vi "CE Measure.vi"(5 "PJVS setup":T1={"PJVS type"=enum."AC-supraVOLTcontrol", "Status Refnum"=refnum, "AC-supraVOLTcontrol"={"IP address:port (0.0.0.0:0000)"="0.0.0.0:0000", "Timeouts"={"TCP Read & Write (ms)"=7000, "Sensors readout"=5000, "PJVS setup"=10000, "Nullmeter readout"=5000, "Multiplexer setup"=3000, "57XX setup"=15000, "Generator setup"=5000, "Synthesizer setup"=3000, "Sampler readout"=10000}, "Simulation mode"=FALSE, "Debug mode"=FALSE}, "NPL bias source"={"DataSocketCluster"={"Server Machine"="CZC", "Client Machine"="localhost", "Data"="P2", "TimeStamp"=0.0, "Count"=1, "Target Process"="General Server"}}, "Manual PJVS"={"PJVS frequency (Hz)"=0.0, "Reference voltages (V)"=[], "File with PJVS voltages"=path ""}, "VTT PJVS"={"some VTT only property"=""}} {"NPL bias source"."DataSocketCluster"."TimeStamp" format="%.2f"}, 6 "AC sync source":T5, 7 "figure prefix ()":string, 8 "error in":errorcluster, 9 "CE measurement":T7={"Signal frequencies (Hz) T"=[1000.0], "Signal amplitudes (V) T"=[0.707], "Sampling frequencies (Hz) T"=[10000000.0], "Record lengths (multiples of periods) T"=[10000.0], "TWM data root directory"=path "", "TWM mreasurements directories"=[], "Calculate RMS from samples"=FALSE, "Algorithm to use"="TWM-WFFT", "Quantity to read"="TWM-WFFT", "Settle down after AC source change (s) T"=1.0, "Skip PJVS setup"=FALSE, "Measurement template file"=path "", "Row of START keyword T"=0, "Row of STOP keyword T"=0, "Measurement template line T"=[], "Switch position T"=[10000.0], "FR fit mat file T"=path "", "Recalculate-skip already calculated"=FALSE} {"Switch position T" format="%#_3p"; "Record lengths (multiples of periods) T" format="%#_3p"; "Sampling frequencies (Hz) T" format="%#_3p"; "Signal amplitudes (V) T" format="%#_3p"; "Signal frequencies (Hz) T" format="%#_3p"}, 10 "AC Source":T5, 11 "Common properties":T8={"Measurement status ref"=refnum, "TWM Status ref"=refnum, "Abort ref"=refnum, "Skip waiting ref"=refnum, "GNU Octave path"=path "C:/Program Files/GNU Octave/Octave-6.2.0/mingw64/bin", "TWM+QWTB path"=path "C:/Users/labina/Desktop/TWM-1.8.7.0-full/octprog", "lvlib path"=path "D:/martin/WAC/WACsw - github/control_software/Filter function meter/external libraries/GOLPI 0.7.3.1 source distribution LV 20.0 32 bit/lv_proc.dll", "TWM pipe"="\\\\.\\pipe\\TWM:server", "PJVS status ref"=refnum, "WAC path"=path ""}) -> (0 "error out":errorcluster)   [LabVIEW 2020]
doc: "Main VI to run cable error measurement. Setup devices, run loop for all freuencies, stop devices."
uses:
  General AC source/Type definitions/AC Source.ctl
  General AC source/Type definitions/AC Source type.ctl
  Utilities/Type definitions/Common properties.ctl
  Type definitions/CE measurement.ctl
  <vilib>/Utility/NIReport.llb/NI_report.lvclass
  General PJVS driver/Type definitions/PJVS.ctl
  General PJVS driver/Type definitions/PJVS Type.ctl
  external libraries/acsvcontrol-driver/Public/Type Definitions/Timeouts.ctl
  external libraries/JV modified NPL Bias source/DataSocketCluster external.ctl
  <vilib>/Utility/error.llb/DialogType.ctl
  external libraries/TWM-1.8.7.0-client/TWM Client.lvlib
  external libraries/acsvcontrol-driver/ACSVcontrol-driver.lvlib
panel:
  out "NI_report":refnum<class "NI_report.lvclass">
  out "previous TWM result value":dbl
  out "previous AC source amplitude":dbl=nan format="%#_13g"
  out "previous AC source frequency":dbl=nan format="%#_13g"
  out "figure reference out":refnum<vi>
  out "TWM handle":i32
  out "figure queue":refnum<queue>
  out "graph x axis":dbl[](array[numeric])
  out "graph y axis":dbl[](array[numeric])
  out "ratio chart":cluster{dbl[], dbl[]}(graph)
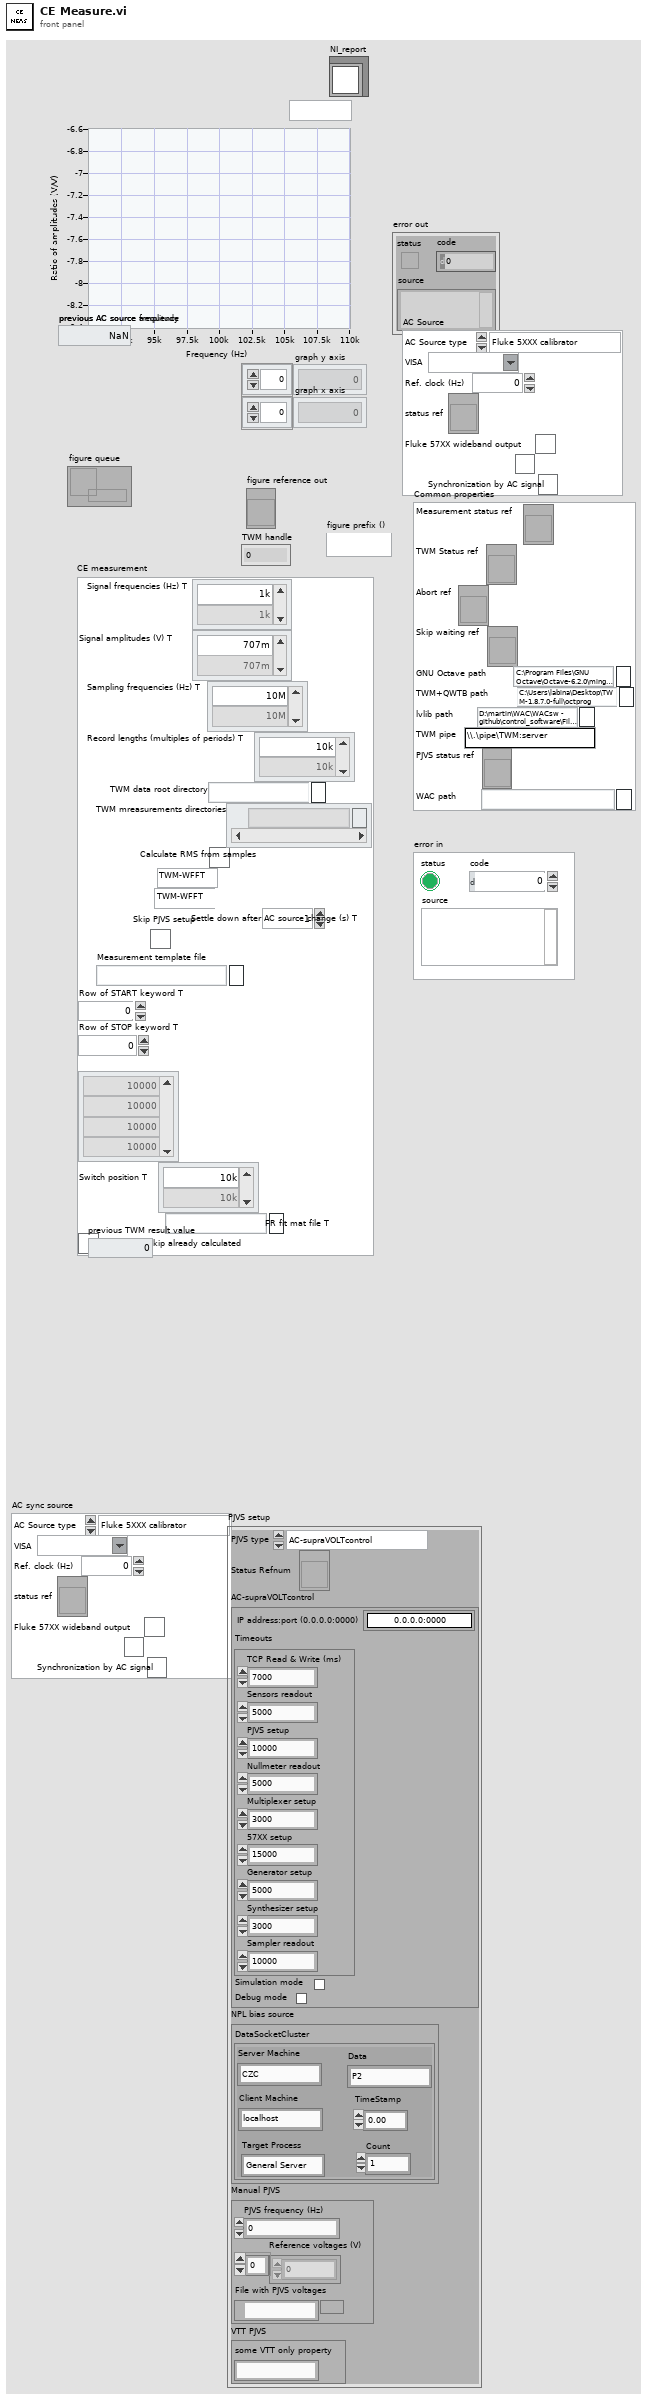
[diagram p1: front panel]
types:
  T1 = typedef "PJVS.ctl" = cluster{"PJVS type":T2, "Status Refnum":refnum<vi>, "AC-supraVOLTcontrol":cluster{"IP address:port (0.0.0.0:0000)":string, "Timeouts":T3, "Simulation mode":bool, "Debug mode":bool}, "NPL bias source":cluster{"DataSocketCluster":T4}, "Manual PJVS":cluster{"PJVS frequency (Hz)":dbl, "Reference voltages (V)":dbl[], "File with PJVS voltages":path}, "VTT PJVS":cluster{"some VTT only property":string}}
  T2 = typedef "PJVS Type.ctl" = enum16{"AC-supraVOLTcontrol", "JV modified NPL bias control", "Manual PJVS", "VTT PJVS"}
  T3 = typedef "ACSVcontrol-driver.lvlib/Timeouts.ctl" = cluster{"TCP Read & Write (ms)":i32, "Sensors readout":i32, "PJVS setup":i32, "Nullmeter readout":i32, "Multiplexer setup":i32, "57XX setup":i32, "Generator setup":i32, "Synthesizer setup":i32, "Sampler readout":i32}
  T4 = typedef "DataSocketCluster external.ctl" = cluster{"Server Machine":string, "Client Machine":string, "Data":string, "TimeStamp":dbl, "Count":i32, "Target Process":string}
  T5 = typedef "AC Source.ctl" = cluster{"AC Source type":T6, "VISA":refnum<visa-resource-name>, "Ref. clock (Hz)":dbl, "status ref":refnum<vi>, "Fluke 57XX wideband output":bool, "Fluke 57XX ignore errors":bool, "Synchronization by AC signal":bool}
  T6 = typedef "AC Source type.ctl" = enum16{"Fluke 5XXX calibrator", "Tektronix AFG3000 series", "dummy", "Agilent 331xxA to 332xxA", "Agilent 335xxA to 336xxA"}
  T7 = typedef "CE measurement.ctl" = cluster{"Signal frequencies (Hz) T":dbl[], "Signal amplitudes (V) T":dbl[], "Sampling frequencies (Hz) T":dbl[], "Record lengths (multiples of periods) T":dbl[], "TWM data root directory":path, "TWM mreasurements directories":path[], "Calculate RMS from samples":bool, "Algorithm to use":string, "Quantity to read":string, "Settle down after AC source change (s) T":dbl, "Skip PJVS setup":bool, "Measurement template file":path, "Row of START keyword T":i32, "Row of STOP keyword T":i32, "Measurement template line T":i32[], "Switch position T":dbl[], "FR fit mat file T":path, "Recalculate-skip already calculated":bool}
  T8 = typedef "Common properties.ctl" = cluster{"Measurement status ref":refnum<vi>, "TWM Status ref":refnum<vi>, "Abort ref":refnum<vi>, "Skip waiting ref":refnum<vi>, "GNU Octave path":path, "TWM+QWTB path":path, "lvlib path":path, "TWM pipe":string, "PJVS status ref":refnum<vi>, "WAC path":path}
  T9 = typedef "DialogType.ctl" = u16
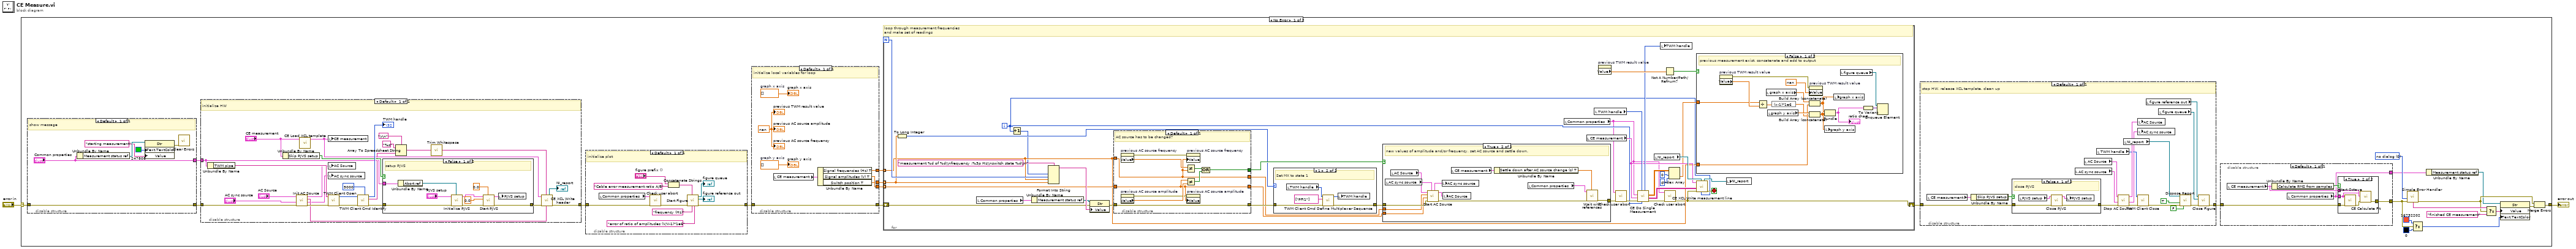
[diagram p0: block diagram]
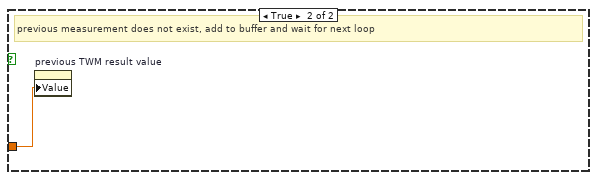
[diagram p3: hidden frame]
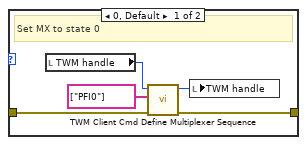
[diagram p5: hidden frame]
diagram:
  n1 = case shown="No Error" "error in" {
    selector: "error in" -> [w3 w206]
    tunnel: [w10 w206] -> w2
    frame No Error {
      w12 = T9 0 items=["no dialog", "OK message", "continue or stop message", "OK message + warnings", "continue/stop + warnings"] ("type of dialog (OK msg:1)")
      n2 = disable-structure shown="Default" {
        disable-tunnel: w3 -> [w58]
        disable-tunnel: [w58] -> w24
        disable-tunnel: ["Common properties"] -> w23
        frame Enabled {
          # "show message"
          n3 = Unbundle By Name("Common properties") -> ("Measurement status ref"=w61:refnum<vi>)
          n4 = property class="Str"(reference=w61, "Text.TextColor"=u32 247808 ("Text.Text Colors:Text Color"), "Value"="starting measurement") -> (error out=w62:errorcluster)  [unwired: 1 in, 1 out]
          n5 = call <vilib>:"Clear Errors.vi"("error in (no error)"=w62) -> ()  [unwired: 5 in, 2 out]
        }
      }
      n6 = disable-structure shown="Default" {
        disable-tunnel: [w180] -> w26
        disable-tunnel: w24 -> [w186]
        disable-tunnel: w23 -> [w170]
        frame Enabled {
          # "initialize HW"
          n7 = Unbundle By Name(w170) -> ("TWM pipe"=w189:string)
          n8 = Unbundle By Name("CE measurement") -> ("Skip PJVS setup"=w185:bool)
          n9 = call "Init AC Source.vi"("error in (no error)"=w186, "AC sync source"="AC sync source", "AC source"="AC Source") -> ("error out"=w190:errorcluster, "AC sync source out"=w171:T5, "Init status"=w179:string, "AC source out"=w187:T5)  [unwired: 5 in]
          n10 = call "CE Load XCL template.vi"("CE measurement"="CE measurement") -> ("CE measurement out"=w182:T7)  [unwired: 9 in, 1 out]
          n11 = local write "CE measurement"(w182) -> ()
          n12 = local write "AC Source"(w187) -> ()
          n13 = local write "AC sync source"(w171) -> ()
          n14 = call "TWM Client Open.vi"("error in"=w190, "pipe name"=w189) -> ("error out"=w193:errorcluster, "handle out"=w194:i32)  [unwired: 8 in]
          n15 = call "TWM Client Cmd Identify.vi"("timeout [ms]"=5000, "error in"=w193, "handle"=w194) -> ("error out"=w184:errorcluster, "channel idns"=w176:string[], "handle out"=→"TWM handle":i32)  [unwired: 5 in, 1 out]
          n16 = case shown="False" w185 {
            tunnel: [w200 w205] -> w181
            tunnel: w184 -> [w201 w205]
            tunnel: w170 -> [w197 _]
            frame False {
              # "setup PJVS"
              n17 = Unbundle By Name(w197) -> ("Abort ref"=w196:refnum<vi>)
              n18 = call "Initialize PJVS.vi"("Abort Refnum"=w196, "error in (no error)"=w201, "PJVS setup"="PJVS setup") -> ("error out"=w202:errorcluster, "PJVS setup out"=w198:T1)  [unwired: 7 in]
              n19 = call "Start PJVS.vi"("Requested PJVS frequency (Hz)"=0.0, "error in (pass through)"=w202, "Maximal signal amplitude (V)"=0.0, "PJVS setup"=w198) -> ("error out"=w200:errorcluster, "PJVS setup out"=w195:T1)  [unwired: 3 in, 3 out]
              n20 = local write "PJVS setup"(w195) -> ()
            }
            frame True {
            }
          }
          n21 = Array To Spreadsheet String(delimiter (Tab)="\r\n", array=w176, 3:"%s" ("format string")) -> (spreadsheet string=w178:string)
          n22 = call <vilib>:"Trim Whitespace.vi"("string"=w178) -> ("trimmed string"=w174:string)  [unwired: 1 in]
          n23 = call "CE XCL Write header.vi"("AC source idn"=w179, "Digitizer idn"=w174, "error in (no error)"=w181, "CE measurement"=w182) -> ("error out"=w180:errorcluster, "NI_report out"=→"NI_report":refnum<class "NI_report.lvclass">)  [unwired: 6 in]
        }
      }
      n24 = disable-structure shown="Default" {
        disable-tunnel: w26 -> [w56]
        disable-tunnel: [w46] -> w22
        frame Enabled {
          # "initialize plot"
          n25 = local read "Common properties"() -> (w51:T8)
          n26 = call "Check user abort.vi"("error in (no error)"=w56, "Common properties"=w51) -> ("error out"=w55:errorcluster)  [unwired: 9 in]
          n27 = Concatenate Strings("figure prefix ()", "Cable error measurement ratio A/B" ("Plot name (sampled signal)")) -> (w47:string)
          n28 = call "Start Figure.vi"("Y scale label (amplitude (V))"="error of ratio of amplitudes (V/V-1)*1e6", "X scale label (time(s))"="frequency (Hz)", "Plot name (sampled signal)"=w47, "error in (no error)"=w55) -> ("error out"=w46:errorcluster, "figure reference out"=→"figure reference out":refnum<vi>, "queue out"=→"figure queue":refnum<queue>)  [unwired: 5 in]
        }
      }
      n29 = disable-structure shown="Default" {
        disable-tunnel: [w45] -> w21
        disable-tunnel: w22 -> [w45]
        disable-tunnel: [w40] -> w6
        disable-tunnel: [w39] -> w5
        disable-tunnel: [w38] -> w4
        frame Enabled {
          w42 = dbl[] []  # graph y axis
          w43 = dbl[] []  # graph x axis
          w44 = nan ("previous TWM result value")
          # "initialize local variables for loop"
          n30 = local read "CE measurement"() -> (w41:T7)
          n31 = Unbundle By Name(w41) -> ("Signal frequencies (Hz) T"=w40:dbl[], "Signal amplitudes (V) T"=w39:dbl[], "Switch position T"=w38:dbl[])
          "previous AC source frequency" <- w44
          "previous AC source amplitude" <- w44
          "previous TWM result value" <- w44
          "graph y axis" <- w42
          "graph x axis" <- w43
        }
      }
      n32 = for {
        N -> [w96]
        shift-right: [w64] -> w25
        shift-left: w21 -> [w95]
        tunnel: w6 -> [w72] mode=indexing
        tunnel: w5 -> [w84] mode=indexing
        tunnel: w4 -> [w81] mode=indexing
        i -> [w67]
        stop <- w75 stop-if-true
        # "loop through measurement frequencies\nand make set of readings"
        n33 = To Long Integer(number=w81) -> (32bit integer=w80:i32)
        n34 = local read "Common properties"() -> (w93:T8)
        n35 = Increment(x=w67) -> (x+1=w66:i32)
        n36 = Unbundle By Name(w93) -> ("Measurement status ref"=w94:refnum<vi>)
        n37 = Format Into String(format string="measurement %d of %d\\nfrequency :%3p Hz\\nswitch state %d\\n", w66, w96, w72, w81) -> (resulting string=w97:string)  [unwired: 2 in, 1 out]
        n38 = property class="Str"(reference=w94, error in=w95, "Value"=w97) -> (error out=w87:errorcluster)  [unwired: 1 out]
        n39 = disable-structure shown="Default" {
          disable-tunnel: w84 -> [w100]
          disable-tunnel: w72 -> [w99]
          disable-tunnel: [w106] -> w85
          disable-tunnel: w87 -> [w106]
          disable-tunnel: [w103] -> w88
          disable-tunnel: [w100] -> w83
          disable-tunnel: [w99] -> w82
          frame Enabled {
            # "AC source has to be changed?"
            n40 = property on="previous AC source frequency" class="DigNum (strict)"() -> (error out=w101:errorcluster, "Value"=w108:dbl)  [unwired: 2 in, 1 out]
            n41 = property on="previous AC source amplitude" class="DigNum (strict)"() -> (error out=w102:errorcluster, "Value"=w107:dbl)  [unwired: 2 in, 1 out]
            n42 = Not Equal?(x=w108, y=w99) -> (x != y?=w104:bool)
            n43 = Not Equal?(x=w100, y=w107) -> (x != y?=w105:bool)
            n44 = property on="previous AC source frequency" class="DigNum (strict)"(error in=w101, "Value"=w99) -> ()  [unwired: 1 in, 2 out]
            n45 = property on="previous AC source amplitude" class="DigNum (strict)"(error in=w102, "Value"=w100) -> ()  [unwired: 1 in, 2 out]
            n46 = Compound Arithmetic op=OR(w104, w105) -> (w103:bool)
          }
        }
        n47 = case shown="1" w80 {
          tunnel: w85 -> [w138 w143]
          tunnel: [w137 w142] -> w86
          frame 0, Default {
            # "Set MX to state 0"
            n48 = local read "TWM handle"() -> (w140:i32)
            n49 = call "TWM Client Cmd Define Multiplexer Sequence.vi"("error in"=w138, "sequence item strings"=string[] ["PFI0"], "handle"=w140) -> ("error out"=w137:errorcluster, "handle out"=w141:i32)  [unwired: 7 in]
            n50 = local write "TWM handle"(w141) -> ()
          }
          frame 1 {
            # "Set MX to state 1"
            n51 = local read "TWM handle"() -> (w145:i32)
            n52 = call "TWM Client Cmd Define Multiplexer Sequence.vi"("error in"=w143, "sequence item strings"=string[] ["PFI1"], "handle"=w145) -> ("error out"=w142:errorcluster, "handle out"=w146:i32)  [unwired: 7 in]
            n53 = local write "TWM handle"(w146) -> ()
          }
        }
        n54 = case shown="True" w88 {
          tunnel: [w124 w128] -> w79
          tunnel: w86 -> [w124 w136]
          tunnel: w83 -> [_ w135]
          tunnel: w82 -> [_ w134]
          frame False {
            # "no change of AC source"
          }
          frame True {
            # "new values of amplitude and/or frequency, set AC source and settle down."
            n55 = local read "AC sync source"() -> (w130:T5)
            n56 = local read "AC Source"() -> (w133:T5)
            n57 = call "Start AC Source.vi"("AC sync source"=w130, "error in (no error)"=w136, "Signal amplitude (V)"=w135, "Signal frequency  (Hz)"=w134, "AC source"=w133) -> ("error out"=w127:errorcluster, "AC source out"=w132:T5, "AC sync source out"=w129:T5)  [unwired: 3 in, 1 out]
            n58 = local write "AC sync source"(w129) -> ()
            n59 = local write "AC Source"(w132) -> ()
            n60 = local read "CE measurement"() -> (w131:T7)
            n61 = Unbundle By Name(w131) -> ("Settle down after AC source change (s) T"=w126:dbl)
            n62 = local read "Common properties"() -> (w125:T8)
            n63 = call "Wait with references.vi"("seconds to wait (1)"=w126, "error in (no error)"=w127, "Common properties"=w125) -> ("error out"=w128:errorcluster)  [unwired: 8 in]
          }
        }
        n64 = local read "Common properties"() -> (w63:T8)
        n65 = local read "CE measurement"() -> (w74:T7)
        n66 = local read "TWM handle"() -> (w89:i32)
        n67 = property on="previous TWM result value" class="DigNum (strict)"() -> ("Value"=w91:dbl)  [unwired: 2 in, 2 out]
        n68 = call "Check user abort.vi"("error in (no error)"=w79, "Common properties"=w63) -> ("error out"=w78:errorcluster)  [unwired: 9 in]
        n69 = call "CE Do Single Measurement.vi"("Iteration index"=w67, "TWM handle in"=w89, "error in (no error)"=w78, "CE measurement"=w74, "Common properties"=w63) -> ("error out"=w65:errorcluster, "TWM result as string"=w73:string[][], "TWM result as number"=w71:dbl[][], "TWM handle out"=w90:i32)  [unwired: 3 in]
        n70 = local read "NI_report"() -> (w77:refnum<class "NI_report.lvclass">)
        n71 = local write "TWM handle"(w90) -> ()
        n72 = Not A Number/Path/Refnum?(number/path/refnum=w91) -> (NaN/Path/Refnum?=w92:bool)
        n73 = call "Check user abort.vi"("error in (no error)"=w65, "Common properties"=w63) -> ("error out"=w64:errorcluster)  [unwired: 9 in]
        n74 = Index Array(array=w71, index (row)=0, index (col)=0 ("disabled index (col)")) -> (element=w68:dbl)
        n75 = case shown="False" w92 {
          tunnel: w72 -> [w116 _]
          tunnel: w68 -> [w111 w123]
          frame False {
            # "previous measurement exist, concatenate and add to output"
            n76 = property on="previous TWM result value" class="DigNum (strict)"() -> (error out=w113:errorcluster, "Value"=w114:dbl)  [unwired: 2 in, 1 out]
            n77 = Divide(x=w111, y=w114) -> (x/y=w109:dbl)
            n78 = local read "graph x axis"() -> (w120:dbl[])
            n79 = local read "graph y axis"() -> (w118:dbl[])
            n80 = expression code="(x-1)*1e6"(w109) -> (w110:dbl)
            n81 = property on="previous TWM result value" class="DigNum (strict)"(error in=w113, "Value"=nan ("previous TWM result value")) -> ()  [unwired: 1 in, 2 out]
            n82 = Build Array (concatenate)(w120, w116) -> (w121:dbl[])
            n83 = Build Array (concatenate)(w118, w110) -> (w119:dbl[])
            n84 = Bundle(w121, w119) -> (w112:cluster{dbl[], dbl[]})  [unwired: 1 in]
            "ratio chart" <- w112
            n85 = local write "graph y axis"(w119) -> ()
            n86 = local write "graph x axis"(w121) -> ()
            n87 = local read "figure queue"() -> (w122:refnum<queue>)
            n88 = To Variant(anything=w112) -> (Variant=w117:variant)
            n89 = Enqueue Element(queue=w122, element=w117) -> ()  [unwired: 2 in, 3 out]
          }
          frame True {
            # "previous measurement does not exist, add to buffer and wait for next loop"
            n90 = property on="previous TWM result value" class="DigNum (strict)"("Value"=w123) -> ()  [unwired: 2 in, 2 out]
          }
        }
        n91 = call "CE XCL Write measurement line.vi"("Iteration index"=w67, "report in"=w77, "error in (no error)"=w64, "TWM result as string for XCL"=w73, "CE measurement"=w74) -> ("error out"=w75:errorcluster, "report out"=w76:refnum<class "NI_report.lvclass">)  [unwired: 5 in]
        n92 = local write "NI_report"(w76) -> ()
      }
      n93 = disable-structure shown="Default" {
        disable-tunnel: w25 -> [w156]
        disable-tunnel: [w149] -> w9
        frame Enabled {
          # "stop HW, release XCL template, clean up"
          n94 = local read "CE measurement"() -> (w158:T7)
          n95 = Unbundle By Name(w158) -> ("Skip PJVS setup"=w155:bool)
          n96 = case shown="False" w155 {
            tunnel: [w167 w169] -> w157
            tunnel: w156 -> [w168 w169]
            frame False {
              # "close PJVS"
              n97 = local read "PJVS setup"() -> (w166:T1)
              n98 = call "Close PJVS.vi"("error in (pass through)"=w168, "PJVS setup"=w166) -> ("error out"=w167:errorcluster, "PJVS setup out"=w165:T1)  [unwired: 8 in]
              n99 = local write "PJVS setup"(w165) -> ()
            }
            frame True {
            }
          }
          n100 = local read "AC sync source"() -> (w148:T5)
          n101 = local read "AC Source"() -> (w163:T5)
          n102 = local read "TWM handle"() -> (w160:i32)
          n103 = call "Stop AC Source.vi"("error in (no error)"=w157, "AC sync source"=w148, "AC source"=w163) -> ("error out"=w164:errorcluster, "AC sync source out"=w147:T5, "AC source out"=w162:T5)  [unwired: 6 in]
          n104 = local read "NI_report"() -> (w151:refnum<class "NI_report.lvclass">)
          n105 = local write "AC Source"(w162) -> ()
          n106 = local write "AC sync source"(w147) -> ()
          n107 = call "TWM Client Close.vi"("error in"=w164, "handle in"=w160) -> ("error out"=w152:errorcluster)  [unwired: 9 in]
          n108 = local read "figure reference out"() -> (w161:refnum<vi>)
          n109 = local read "figure queue"() -> (w159:refnum<queue>)
          n110 = call-dynamic "Dispose Report.vi"("report in"=w151, "save changes? (F)"=TRUE, "error in (no error)"=w152, "close report? (T)"=FALSE) -> ("error out"=w150:errorcluster)  [unwired: 11 in]
          n111 = call "Close Figure.vi"("error in (passthrough)"=w150, "queue"=w159, "figure reference"=w161) -> ("error out"=w149:errorcluster)  [unwired: 8 in]
        }
      }
      n112 = disable-structure shown="Default" {
        disable-tunnel: w9 -> [w31]
        disable-tunnel: [w30] -> w8
        disable-tunnel: [w27] -> w7
        frame Enabled {
          n113 = local read "CE measurement"() -> (w29:T7)
          n114 = Unbundle By Name(w29) -> ("Calculate RMS from samples"=w28:bool)
          n115 = local read "Common properties"() -> (w27:T8)
          n116 = case shown="True" w28 {
            tunnel: w31 -> [w32 w37]
            tunnel: [w32 w35] -> w30
            tunnel: w29 -> [_ w34]
            tunnel: w27 -> [_ w33]
            frame False {
            }
            frame True {
              n117 = call "Start Octave.vi"("error in (no error)"=w37, "Common properties"=w33) -> ("error out"=w36:errorcluster)  [unwired: 9 in]
              n118 = call "CE Calculate Fit.vi"("error in (no error)"=w36, "CE measurement"=w34, "Common properties"=w33) -> ("error out"=w35:errorcluster)  [unwired: 8 in]
            }
          }
        }
      }
      n119 = call <vilib>:"Simple Error Handler.vi"("type of dialog (OK msg:1)"=w12, "error in (no error)"=w8) -> ("error out"=w16:errorcluster, "message"=w20:string)  [unwired: 3 in, 3 out]
      n120 = Select(t=u32 16732202 ("Text.Text Colors:Text Color"), s=w8, f=u32 0 ("Text.Text Colors:Text Color")) -> (s? t:f=w18:u32)
      n121 = Unbundle By Name(w7) -> ("Measurement status ref"=w15:refnum<vi>)
      n122 = Select(t=w20, s=w16, f="finished CE measurement") -> (s? t:f=w19:string)
      n123 = property class="Str"(reference=w15, "Value"=w19, "Text.TextColor"=w18) -> (error out=w17:errorcluster)  [unwired: 1 in, 1 out]
      n124 = Merge Errors(w16, w17) -> (w10:errorcluster)
    }
    frame Error {
    }
  }
  "error out" <- w2
